vi "Set Filter Interval.vi"(8 "error in":errorcluster, 10 "Int In":sgl=0.1 min=0.1 max=1, 11 "Vaisala in":refnum<class "Vaisala.lvclass">) -> (0 "error out":errorcluster, 2 "Int Out":sgl, 3 "Vaisala out":refnum<class "Vaisala.lvclass">)   [LabVIEW 2014, in "Vaisala Library.lvlib" / "Vaisala.lvclass"]
doc: "Use this command to set the speed at which the latest measurement result is integrated into the humidity and temperature readings. The command affects both analog output and serial line output.\n\nThe range of the input <b>Int </b> is 0.1...1.0.\n\n* 1.0 = No filtering, latest measurement is output without averaging\n* 0.5 = Average of last two measurements\n* 0.1 Average of approximately 16 measurements\n\nThis command will return the new value."
uses:
  Vaisala.lvclass
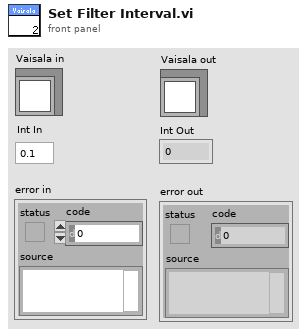
[diagram p1: front panel]
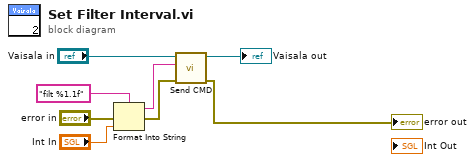
[diagram p0: block diagram]
diagram:
  n1 = Format Into String(format string="filt %1.1f", error in="error in", "Int In") -> (resulting string=w4:string, error out=w3:errorcluster)  [unwired: 1 in]
  n2 = call "Send CMD.vi"("error in"=w3, "CMD In"=w4, "Vaisala in"="Vaisala in") -> ("error out"=→"error out":errorcluster, "Vaisala out"=→"Vaisala out":refnum<class "Vaisala.lvclass">)  [unwired: 7 in]
